vi "Process State Queue.vi"(0 "reference in":refnum<class "Generic Utilities.lvclass">, 5 "error in (no error)":errorcluster) -> (7 "After Command Comments":string, 9 "State History":string[](array[string]), 11 "Additional Options":string, 12 "Timeout":i32, 13 "State Option":string, 14 "reference out":refnum<class "Generic Utilities.lvclass">, 16 "Current State":string, 19 "error out":errorcluster)   [LabVIEW 2020, in "Generic Utilities.lvclass"]
uses:
  Generic Utilities.lvclass
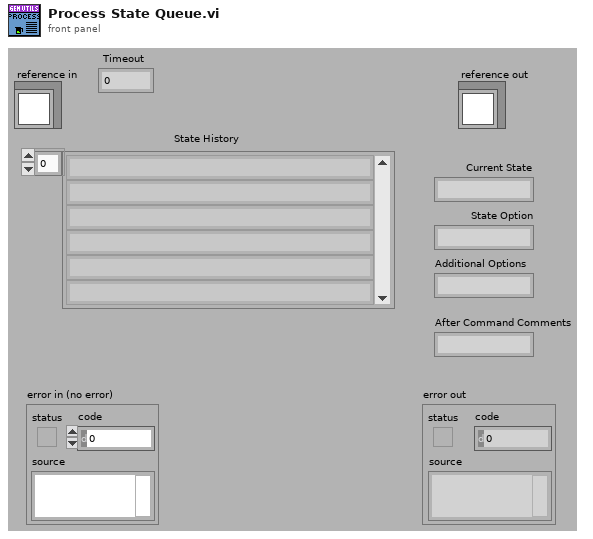
[diagram p1: front panel]
types:
  T1 = typedef "Generic Utilities.lvclass/ObjectAttributesRef.ctl" = refnum<data-value>
  T2 = typedef "Generic Utilities.lvclass/ObjectAttributes.ctl" = cluster{"GUI Parameters":T3, "State Machine Control":cluster{"Timeout":i32, "State Queue":string[], "State History":string[], "State History Length":i32}, "Logging File Path":path, "OBJ not a refnum?":bool, "Timer Start":timestamp, "FP Refnums":T4}
  T3 = typedef "Generic Utilities.lvclass/GUI Parameters.ctl" = cluster{"Application Name":string, "GUI VI Ref":refnum<vi>, "Close Panel?":bool, "Message Window ref":refnum<vi>, "Version #":string}
  T4 = typedef "Generic Utilities.lvclass/FP Refnums.ctl" = cluster{"Panel refnum":refnum<vi>, "Control Labels":string[], "Refnums":refnum<vi>[]}
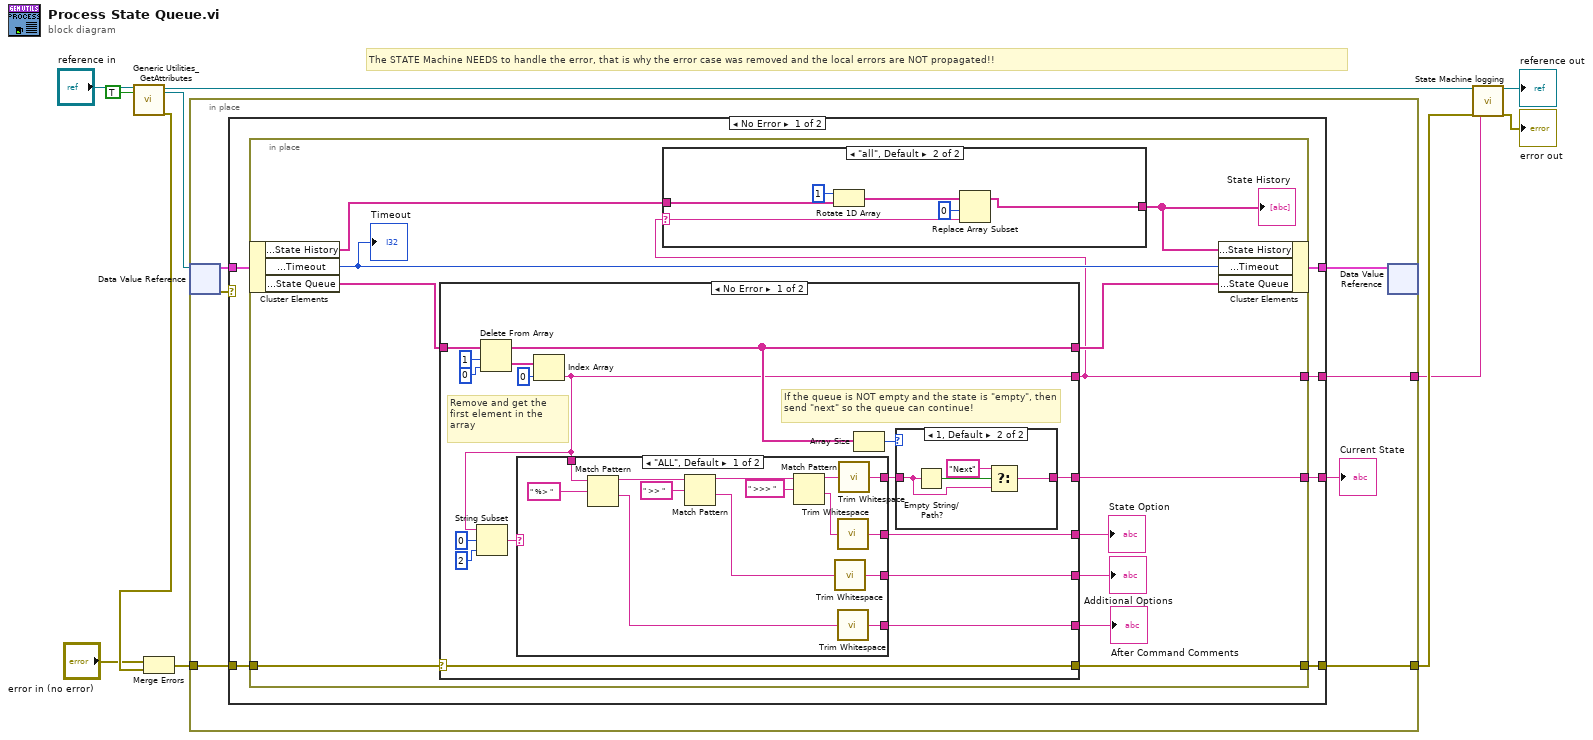
[diagram p0: block diagram]
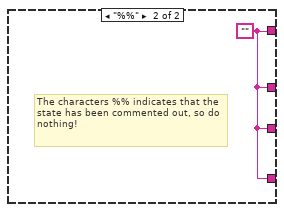
[diagram p3: hidden frame]
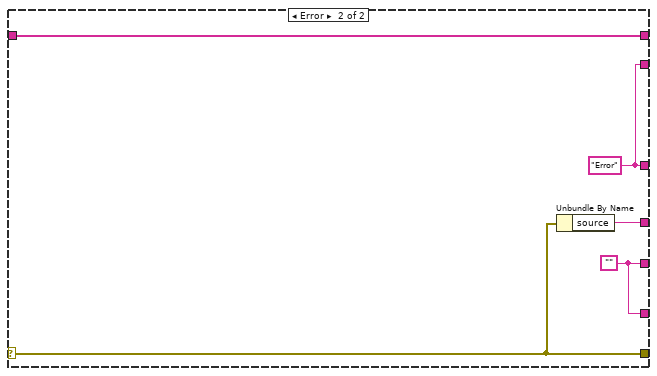
[diagram p5: hidden frame]
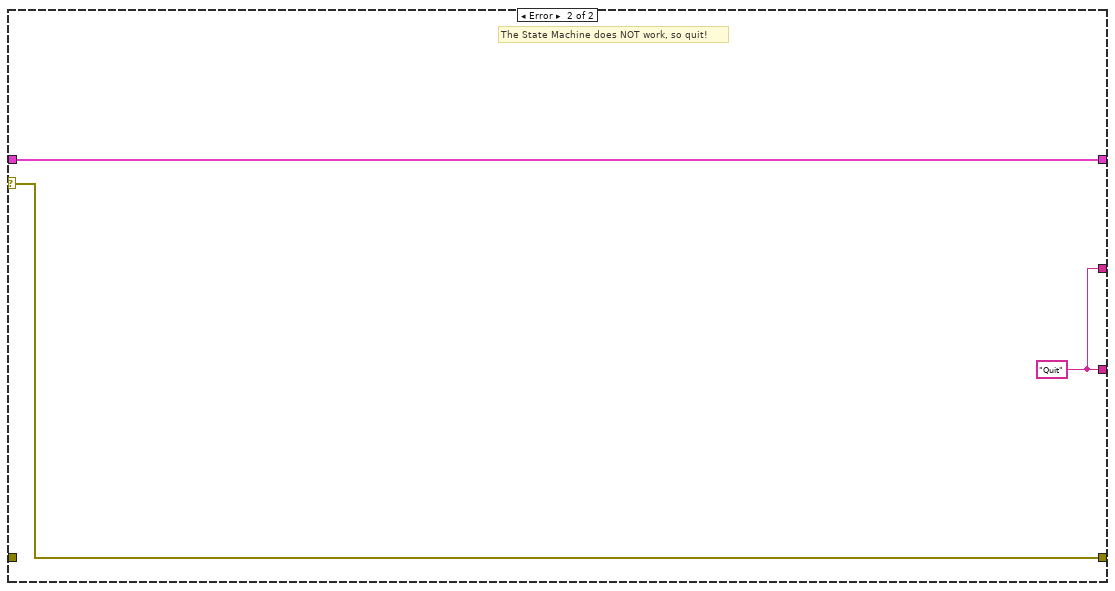
[diagram p6: hidden frame]
diagram:
  # "The STATE Machine NEEDS to handle the error, that is why the error case was removed and the local errors are NOT propagated!!"
  n1 = call "Generic Utilities_GetAttributes.vi"("reference in"="reference in", "return data? (T)"=TRUE) -> ("reference out"=w5:refnum<class "Generic Utilities.lvclass">, "attributes ref"=w10:T1, "error out"=w8:errorcluster)  [unwired: 14 in, 1 out]
  n2 = Merge Errors("error in (no error)", w8) -> (w7:errorcluster)
  n3 = in-place {
    in-place-border: w7 -> [w16]
    in-place-border: [w15] -> w3
    in-place-border: [w12] -> w2
    n4 = in-place-dvr #1(w10) -> (w17:T2, w14:errorcluster)
    n5 = case shown="No Error" w14 {
      selector: w14 -> [_ w88]
      tunnel: [w24 w87] -> w18
      tunnel: w17 -> [w23 w87]
      tunnel: w16 -> [w22 _]
      tunnel: [w21 w88] -> w15
      tunnel: [w20 w86] -> w13
      tunnel: [w19 w86] -> w12
      frame No Error {
        n6 = in-place {
          in-place-border: [w34] -> w21
          in-place-border: w22 -> [w28]
          in-place-border: [w27] -> w20
          in-place-border: [w26] -> w19
          n7 = in-place-cluster #2(w23) -> ("State Machine Control.State History"=w31:string[], "State Machine Control.Timeout"=w29:i32, "State Machine Control.State Queue"=w36:string[])
          "Timeout" <- w29
          n8 = case shown="No Error" w28 {
            selector: w28 -> [w55 w83]
            tunnel: w36 -> [w60 w85]
            tunnel: [w49 w85] -> w35
            tunnel: [w51 w84] -> w27
            tunnel: [w55 w83] -> w34
            tunnel: [w54 w82] -> w32
            tunnel: [w53 w81] -> w33
            tunnel: [w48 w84] -> w26
            tunnel: [w44 w81] -> w25
            frame No Error {
              # "Remove and get the first element in the array"
              # "If the queue is NOT empty and the state is \"empty\", then send \"next\" so the queue can continue!"
              n9 = Delete From Array(array=w60, length=1, index=0) -> (deleted portion=w57:string[], array with subset deleted=w49:string[])
              n10 = Index Array(array=w57, index=0) -> (element=w48:string)
              n11 = String Subset(string=w48, offset (0)=0, length (rest)=2 ("length (rest)")) -> (substring=w45:string)
              n12 = case shown="\"ALL\", Default" w45 {
                tunnel: [w71 w75] -> w54
                tunnel: [w68 w75] -> w53
                tunnel: [w67 w75] -> w52
                tunnel: w48 -> [w65 _]
                tunnel: [w61 w75] -> w44
                frame "ALL", Default {
                  n13 = Match Pattern(string=w65, regular expression=" %> ") -> (before substring=w63:string, after substring=w62:string)  [unwired: 1 in, 2 out]
                  n14 = Match Pattern(string=w63, regular expression=" >> ") -> (before substring=w69:string, after substring=w66:string)  [unwired: 1 in, 2 out]
                  n15 = Match Pattern(string=w69, regular expression=" >>> ") -> (before substring=w73:string, after substring=w74:string)  [unwired: 1 in, 2 out]
                  n16 = call <vilib>:"Trim Whitespace.vi"("string"=w66) -> ("trimmed string"=w68:string)  [unwired: 1 in]
                  n17 = call <vilib>:"Trim Whitespace.vi"("string"=w74) -> ("trimmed string"=w71:string)  [unwired: 1 in]
                  n18 = call <vilib>:"Trim Whitespace.vi"("string"=w62) -> ("trimmed string"=w61:string)  [unwired: 1 in]
                  n19 = call <vilib>:"Trim Whitespace.vi"("string"=w73) -> ("trimmed string"=w67:string)  [unwired: 1 in]
                }
                frame "%%" {
                  w75 = ""
                  # "The characters %% indicates that the state has been commented out, so do nothing!"
                }
              }
              n20 = Array Size(array=w49) -> (size(s)=w50:i32)
              n21 = case shown="1, Default" w50 {
                tunnel: w52 -> [w76 w78]
                tunnel: [w76 w77] -> w51
                frame 0 {
                }
                frame 1, Default {
                  n22 = Empty String/Path?(string/path=w78) -> (empty?=w79:bool)
                  n23 = Select(t="Next" ("f"), s=w79, f=w78) -> (s? t:f=w77:string)
                }
              }
            }
            frame Error {
              w81 = ""
              w84 = "Error" ("String")
              n24 = Unbundle By Name(w83) -> ("source"=w82:string)
            }
          }
          "State Option" <- w32
          "Additional Options" <- w33
          "After Command Comments" <- w25
          n25 = case shown="\"all\", Default" w26 {
            selector: w26 -> [_ w39]
            tunnel: w31 -> [w37 w43]
            tunnel: [w37 w40] -> w30
            frame "" {
            }
            frame "all", Default {
              n26 = Rotate 1D Array(1:w43, 2:1 ("n")) -> (0:w41:string[])
              n27 = Replace Array Subset(array=w41, new element=w39, index=0) -> (w40:string[])
            }
          }
          "State History" <- w30
          n28 = in-place-cluster #2("State Machine Control.State History"=w30, "State Machine Control.Timeout"=w29, "State Machine Control.State Queue"=w35) -> (w24:T2)
        }
      }
      frame Error {
        w86 = "Quit" ("String")
        # "The State Machine does NOT work, so quit!"
      }
    }
    "Current State" <- w13
    n29 = in-place-dvr #1(w18) -> ()  [unwired: 2 out]
  }
  n30 = call "State Machine logging.vi"("reference in"=w5, "error in (no error)"=w3, "Latest State"=w2) -> ("reference out"=→"reference out":refnum<class "Generic Utilities.lvclass">, "error out"=→"error out":errorcluster)  [unwired: 15 in]
